vi "GDSLvClass_GetClassMembers.vi"(0 "Class Refnum In":refnum<vi>, 1 "VINames":string[](array[string]), 5 "error in (no error)":errorcluster) -> (14 "Class Refnum Out":refnum<vi>, 15 "Members":T1[](array[typedef]), 16 "MethodAbsolutePath":path[](array[path]), 17 "Found":bool, 19 "error out":errorcluster)   [LabVIEW 2020]
uses:
  GDSLvClass_ClassMethodInfo.ctl
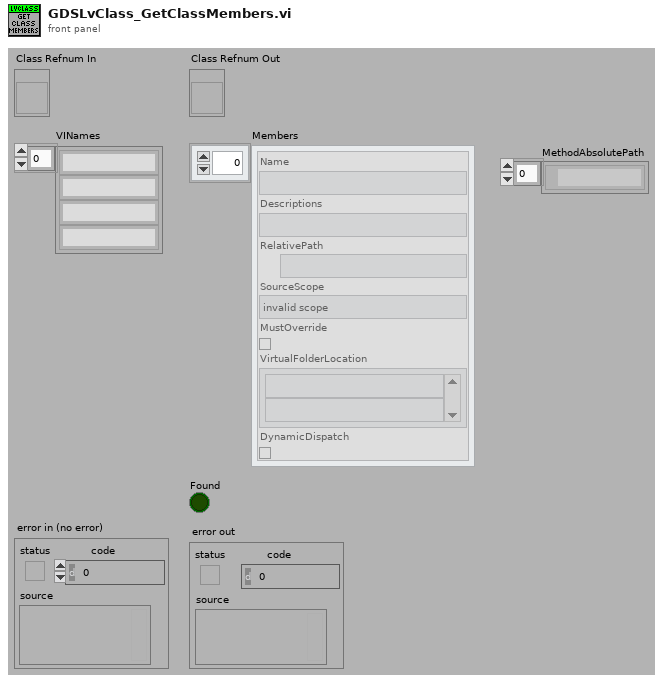
[diagram p1: front panel]
types:
  T1 = typedef "GDSLvClass_ClassMethodInfo.ctl" = cluster{"Name":string, "Descriptions":string, "RelativePath":path, "SourceScope":enum32{"invalid scope", "public", "private", "protected", "community"}, "MustOverride":bool, "VirtualFolderLocation":string[], "DynamicDispatch":bool}
  T2 = enum32{"invalid scope", "public", "private", "protected", "community"}
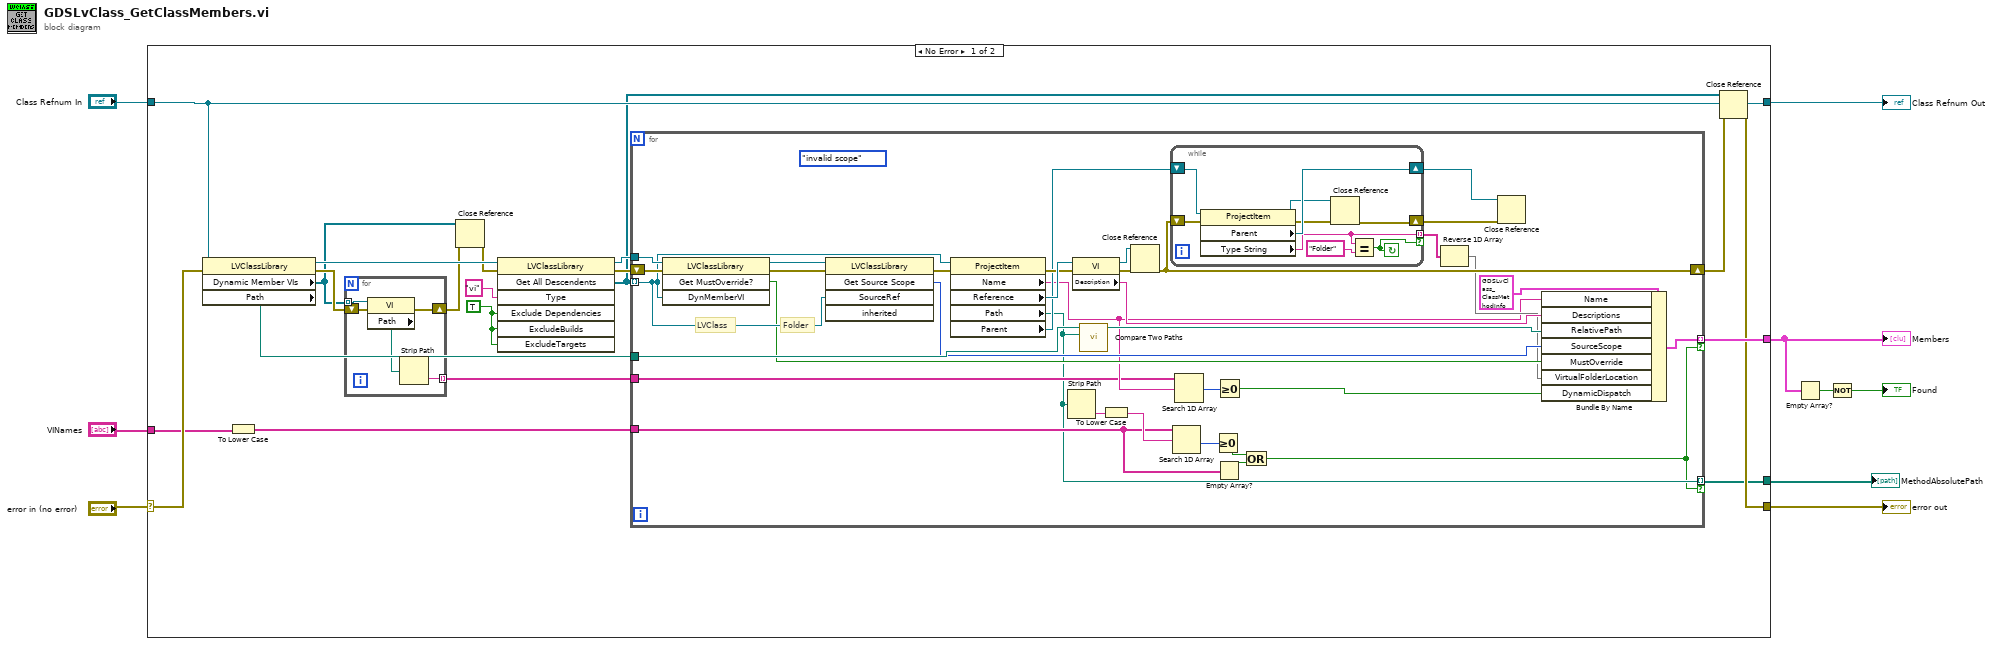
[diagram p0: block diagram]
diagram:
  n1 = case shown="No Error" "error in (no error)" {
    selector: "error in (no error)" -> [w22 w80]
    tunnel: [w13 w80] -> w8
    tunnel: "Class Refnum In" -> [w19 w79]
    tunnel: [w19 w79] -> w6
    tunnel: "VINames" -> [w12 _]
    tunnel: [w20 _] -> w4
    tunnel: [w10 _] -> w1
    frame No Error {
      w23 = TRUE ("ExcludeDependencies")
      n2 = property class="LVClassLibrary"(reference=w19, error in=w22) -> (reference out=w27:refnum<vi>, error out=w28:errorcluster, "Dynamic Member VIs"=w16:refnum<vi>[], "Path"=w21:path)
      n3 = To Lower Case(string=w12) -> (all lower case string=w11:string[])
      n4 = for {
        tunnel: w16 -> [w34] mode=indexing
        shift-right: [w32] -> w18
        shift-left: w28 -> [w33]
        tunnel: [w30] -> w29 mode=indexing
        n5 = property class="VI"(reference=w34, error in=w33) -> (error out=w32:errorcluster, "Path"=w31:path)  [unwired: 1 out]
        n6 = Strip Path(path=w31) -> (name=w30:string)  [unwired: 1 out]
      }
      n7 = Close Reference(reference=w16, error in (no error)=w18) -> (error out=w17:errorcluster)
      n8 = invoke class="LVClassLibrary" method="Get All Descendents"(reference=w27, error in=w17, "Type"="vi", "Exclude Dependencies"=w23, "ExcludeBuilds"=w23, "ExcludeTargets"=w23) -> (reference out=w26:refnum<vi>, error out=w25:errorcluster, "All Descendents"=w15:refnum<vi>[])  [unwired: 1 in, 4 out]
      n9 = for {
        tunnel: w15 -> [w59] mode=indexing
        shift-right: [w55] -> w14
        shift-left: w25 -> [w64]
        tunnel: w26 -> [w65]
        tunnel: w21 -> [w63]
        tunnel: [w47] -> w20 mode=indexing if=w35
        tunnel: w29 -> [w45]
        tunnel: w11 -> [w39]
        tunnel: [w36] -> w10 mode=indexing if=w35
        (unwired) T2."invalid scope" ("Source Scope:Get")
        # "Folder"
        # "LVClass"
        n10 = invoke class="LVClassLibrary" method="Get MustOverride?"(reference=w65, error in=w64, "DynMemberVI"=w59) -> (reference out=w60:refnum<vi>, error out=w58:errorcluster, "GetMustOverride"=w49:bool)  [unwired: 1 in, 1 out]
        n11 = invoke class="LVClassLibrary" method="Get Source Scope"(reference=w60, error in=w58, "SourceRef"=w59) -> (error out=w57:errorcluster, "GetSourceScope"=w50:T2)  [unwired: 2 in, 3 out]
        n12 = property class="ProjectItem"(reference=w59, error in=w57) -> (error out=w67:errorcluster, "Name"=w46:string, "Reference"=w69:refnum<vi>, "Path"=w36:path, "Parent"=w62:refnum<vi>)  [unwired: 1 out]
        n13 = Strip Path(path=w36) -> (name=w42:string)  [unwired: 1 out]
        n14 = property class="VI"(reference=w69, error in=w67) -> (reference out=w68:refnum<vi>, error out=w66:errorcluster, "Description"=w52:string)
        n15 = call <vilib>:"Compare Two Paths.vi"("Path 2"=w36, "Path 1"=w63) -> ("Relative Path from 1 to 2"=w51:path)  [unwired: 6 in, 3 out]
        n16 = To Lower Case(string=w42) -> (all lower case string=w41:string)
        n17 = Close Reference(reference=w68, error in (no error)=w66) -> (error out=w55:errorcluster)
        n18 = while {
          tunnel: [w76] -> w61 mode=indexing if=w74
          shift-right: [w77] -> w56
          shift-left: w62 -> [w78]
          shift-right: [w70] -> w54
          shift-left: w55 -> [w73]
          stop <- w74 continue-if-true
          n19 = property class="ProjectItem"(reference=w78, error in=w73) -> (reference out=w72:refnum<vi>, error out=w71:errorcluster, "Parent"=w77:refnum<vi>, "Type String"=w76:string)
          n20 = Close Reference(reference=w72, error in (no error)=w71) -> (error out=w70:errorcluster)
          n21 = Equal?(x=w76, y="Folder") -> (x = y?=w74:bool)
        }
        n22 = Search 1D Array(1D array=w39, element=w41) -> (index of element=w40:i32)  [unwired: 1 in]
        n23 = Search 1D Array(1D array=w45, element=w46) -> (index of element=w44:i32)  [unwired: 1 in]
        n24 = Greater Or Equal To 0?(x=w40) -> (x >= 0?=w38:bool)
        n25 = Empty Array?(array=w39) -> (empty?=w37:bool)
        n26 = Greater Or Equal To 0?(x=w44) -> (x >= 0?=w43:bool)
        n27 = Or(x=w38, y=w37) -> (x .or. y?=w35:bool)
        n28 = Reverse 1D Array(array=w61) -> (reversed array=w48:string[])
        n29 = Close Reference(reference=w56, error in (no error)=w54) -> ()  [unwired: 1 out]
        n30 = Bundle By Name(cluster=T1 {"Name"="", "Descriptions"="", "RelativePath"=path "", "SourceScope"=enum."invalid scope", "MustOverride"=FALSE, "VirtualFolderLocation"=[], "DynamicDispatch"=FALSE} ("MethodSettings"), "Name"=w46, "Descriptions"=w52, "RelativePath"=w51, "SourceScope"=w50, "MustOverride"=w49, "VirtualFolderLocation"=w48, "DynamicDispatch"=w43) -> (w47:T1)
      }
      n31 = Close Reference(reference=w15, error in (no error)=w14) -> (error out=w13:errorcluster)
    }
    frame Error {
    }
  }
  "Class Refnum Out" <- w6
  "error out" <- w8
  "Members" <- w4
  "MethodAbsolutePath" <- w1
  n32 = Empty Array?(array=w4) -> (empty?=w3:bool)
  n33 = Not(x=w3) -> (.not. x?=→"Found":bool)
